vi "RT-XML-Array.vi"() -> ()   [LabVIEW 2020]
panel:
  out "Array":dbl[][](array[numeric])
  in  "test_set?":bool=TRUE
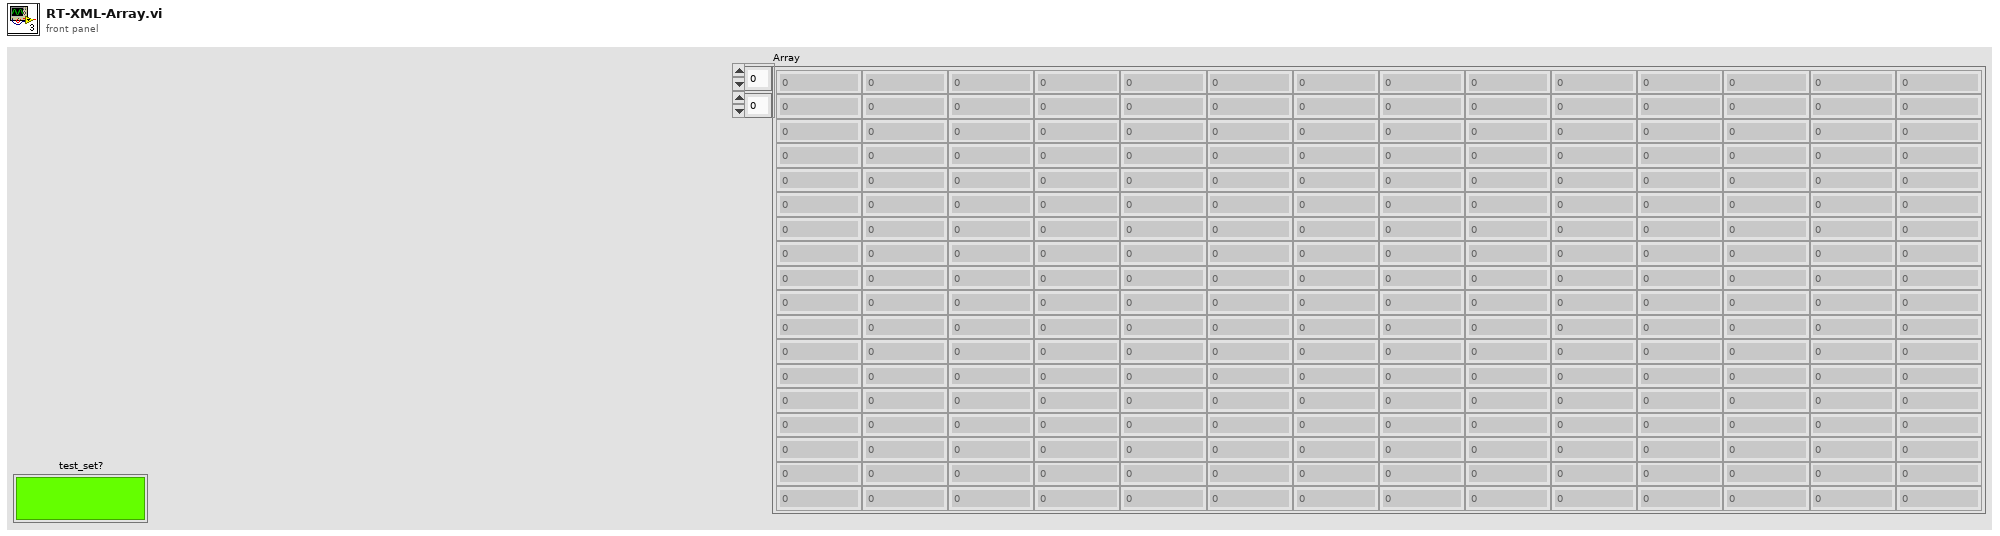
[diagram p1: front panel]
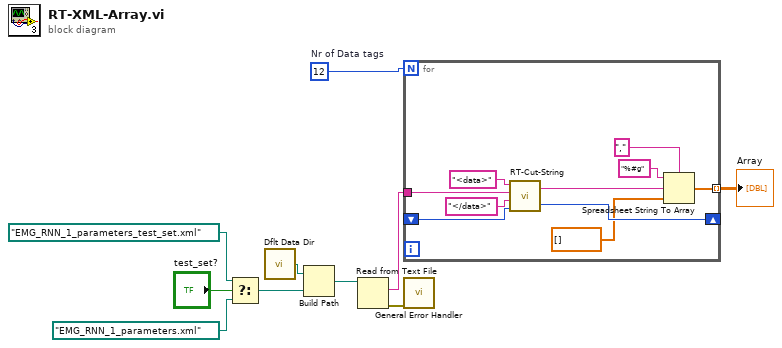
[diagram p0: block diagram]
diagram:
  w1 = 12  # Nr of Data tags
  n1 = Select(t=path "EMG_RNN_1_parameters_test_set.xml" ("name or relative path"), s="test_set?", f=path "EMG_RNN_1_parameters.xml" ("name or relative path")) -> (s? t:f=w5:path)
  n2 = call <vilib>:"Dflt Data Dir.vi"() -> ("App:Default Data Directory"=w10:path)
  n3 = Build Path(base path=w10, name or relative path=w5) -> (appended path=w9:path)
  n4 = Read from Text File(file (use dialog)=w9) -> (text=w8:string, error out=w7:errorcluster)  [unwired: 3 in, 2 out]
  n5 = for {
    N: w1 -> [_]
    tunnel: [w12] -> w2 mode=indexing
    tunnel: w8 -> [w19]
    shift-right: [w16] -> _
    shift-left: _ -> [w17]
    n6 = call "RT-Cut-String.vi"("offset (0)"=w17, "End Cut"="</data>", "Input string"=w19, "Start Cut"="<data>") -> ("offset past match"=w16:i32, "Extracted"=w14:string)
    n7 = Spreadsheet String To Array(delimiter (Tab)="," ("search string/char (-)"), format string="%#g", spreadsheet string=w14, array type (2D Dbl)=dbl[] []) -> (array=w12:dbl[])
  }
  "Array" <- w2
  n8 = call <vilib>:"General Error Handler.vi"("error in (no error)"=w7) -> ()  [unwired: 10 in, 5 out]
